vi "DataPackerDaemon.vi"(5 "Callers (Main VI name)":string, 6 "Request Debug Mode":bool, 7 "DataPacker Queue":refnum<queue>, 8 "MIDAS Sever Port":u16=12345, 9 "MIDAS Server":string="my_midas_server.domain", 10 "Override Max Event size (Data rate bytes/s). Use MIDAS Default = 0":u32) -> (0 "error out":errorcluster)   [LabVIEW 2018, in "feGEM DataPacker.lvlib"]
uses:
  feGEM DataPacker.lvlib
  DataStructures/GEM_BANK_CLUSTER_typedef.ctl
  DataStructures/GEM_DATA_cluster_typedef.ctl
  DataPacker.lvclass
  StateMachineTypeDef.ctl
  DataPacker.lvclass/DataPacker.ctl
  68ac663a-a3e9-43dc-9a45-1d254e90e99c.vi
  6484ace5-38a1-4ceb-a346-464d1fbc0e14.vi
  794d372c-62f1-4848-9cd1-c1a1182567cd.vi
  DataPacker_ConnectToMIDAS.vi/88b38ab8-c5c0-409b-a7b4-cf79df97607d.vi
  68ac663a-a3e9-43dc-9a45-1d254e90e99c.vi/471e45ec-0d50-43f9-a63f-99eed3aa29fd.vi
  6484ace5-38a1-4ceb-a346-464d1fbc0e14.vi/57d1cc16-e710-4084-af24-8dbbb67df11b.vi
  794d372c-62f1-4848-9cd1-c1a1182567cd.vi/362f5b2f-e8ea-4a71-9028-e325dbdad7c8.vi
  SendStuff/SayThisOnMIDAS.vi
  DataStructures/GEM_BANK_ARRAY_Add_Data.vi
  DataStructures/GEM_BANK_ARRAY_Flatten.vi
  ErrorTypes.ctl
  DataStructures/GEM_BANK_ARRAY.lvclass
  <vilib>/Utility/SystemLogging/NI_SystemLogging.lvlib
panel:
  out "DataPacker Queue\nUsage (%)":dbl(knob) scale=0.0..100.0
  out "CPUMEM LOAD (%)":sgl[](array[numeric])
  out "MIDAS Server IP address":string
  out "error out":errorcluster
  out "Log Client info (non fatal)":errorcluster
  out "stop":bool
  in  "stop 3":bool
  out "% Time Packing (Serializing Queued Data)":dbl(knob) scale=0.0..100.0
  out "Unsent items in queue (at shutdown)":i32
  out "MIDAS Reply":string
  out "# elements in queue":i32
  out "Connection Attempt":u32
  out "MIDAS Addresss":string
  out "MIDAS Port":u16
  out "Frontend Status":string
  out "MIDAS Buffer [for this PC] \nUsage (%)":dbl(knob) scale=0.0..100.0
  out "MIDAS Connection OK":bool
  out "Seconds since last communication with MIDAS":dbl
  out "Last Midas Handling Time (ms)":dbl
  out "Average MIDAS Processing Time (ms)":dbl(knob) scale=1.0..1000.0
  out "System Load Logging Error  (non fatal)":errorcluster
  out "Periodic Task Error (non fatal)":errorcluster
  out "This Computer Name":string
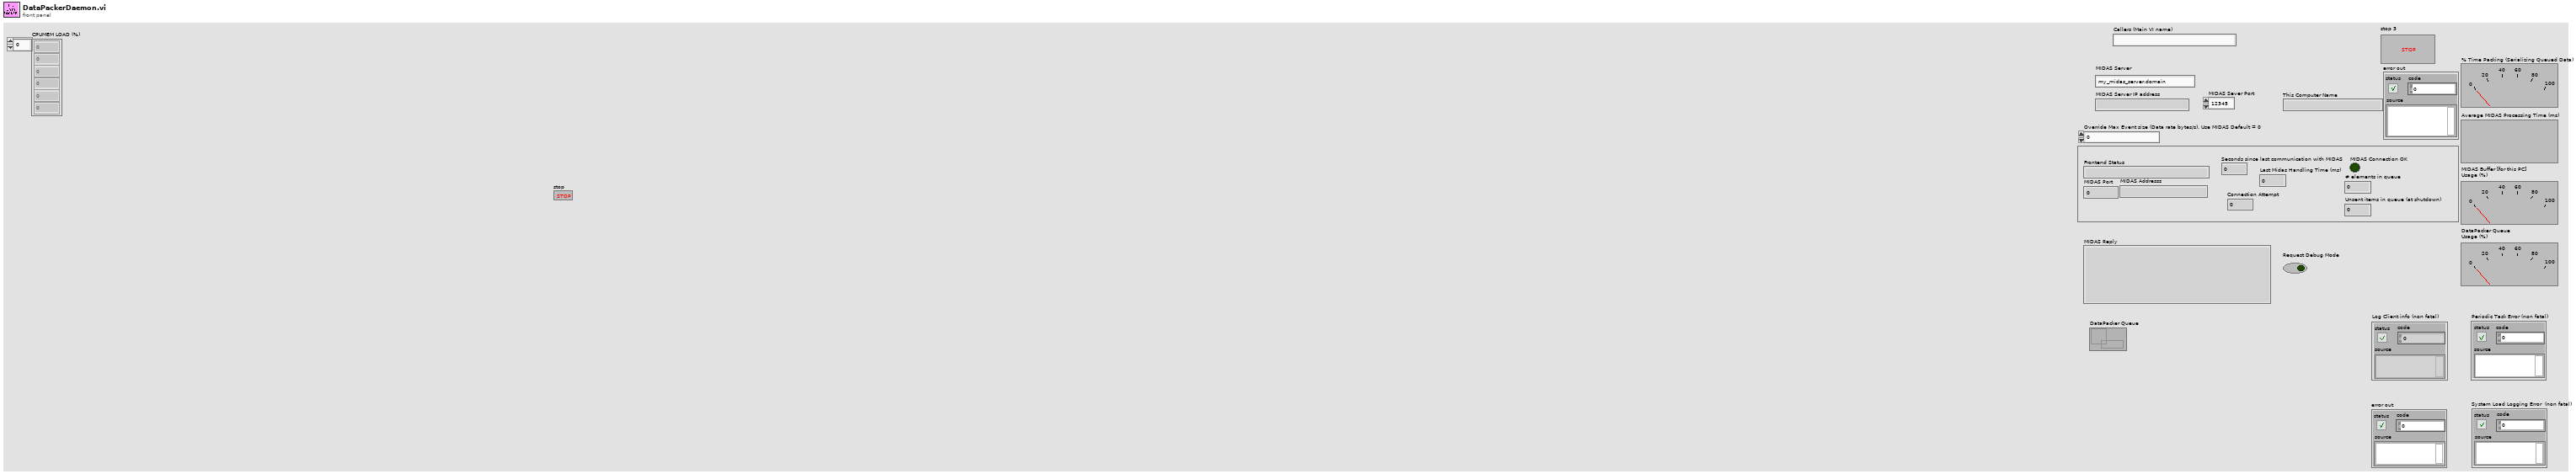
[diagram p1: front panel]
types:
  T1 = typedef "feGEM DataPacker.lvlib/StateMachineTypeDef.ctl" = enum16{"Setup", "Setup SSH", "Connect To Midas", "Get And Set Event Size", "Re-initialise", "Sleep", "BundleDataInQueue", "SerializeBundle", "SendData", "Shutdown", "HandleErrorStates"}
  T2 = typedef "feGEM DataPacker.lvlib/ErrorTypes.ctl" = i32
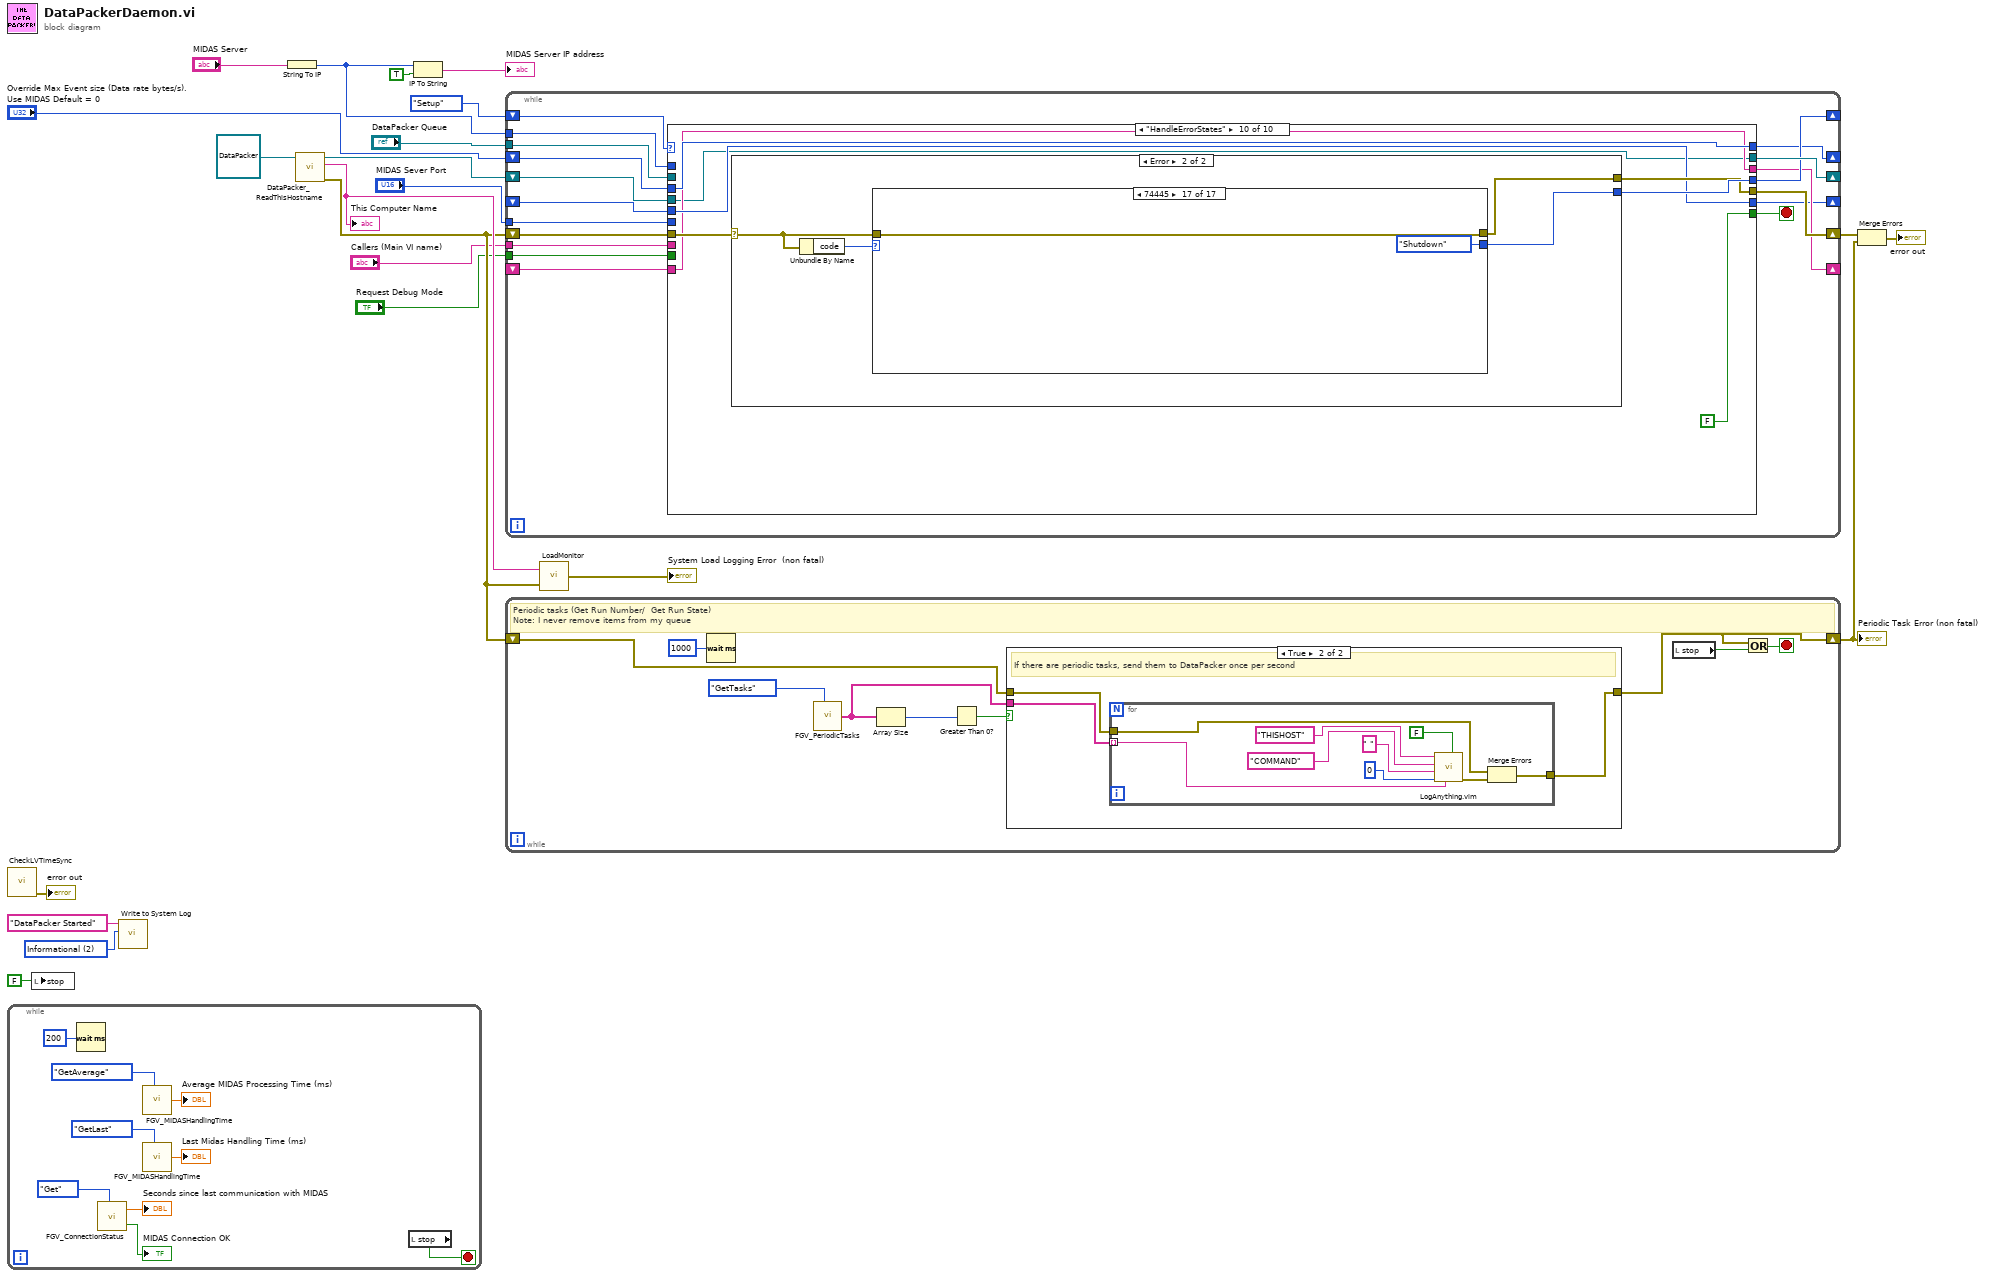
[diagram p0: block diagram]
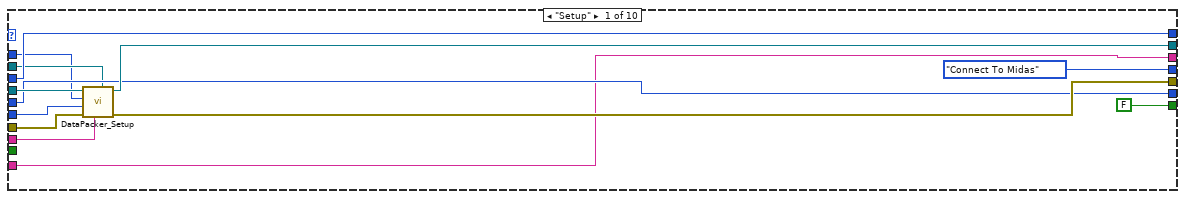
[diagram p2: hidden frame]
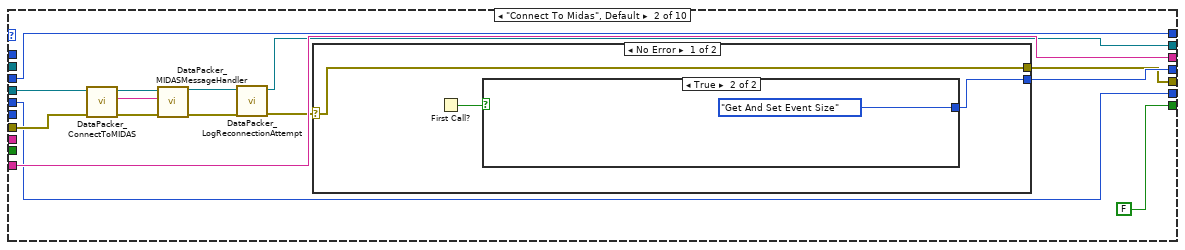
[diagram p3: hidden frame]
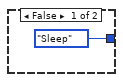
[diagram p4: hidden frame]
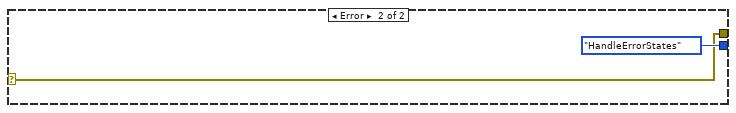
[diagram p5: hidden frame]
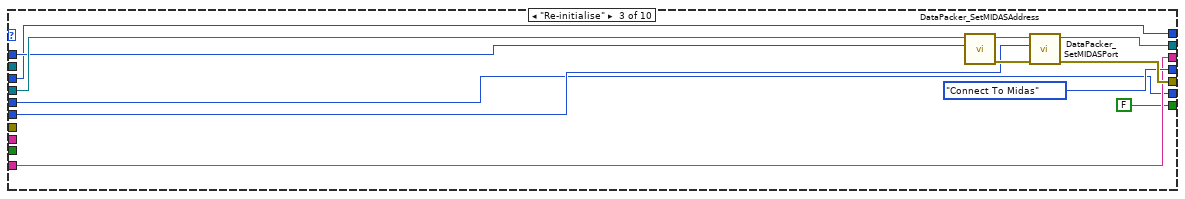
[diagram p6: hidden frame]
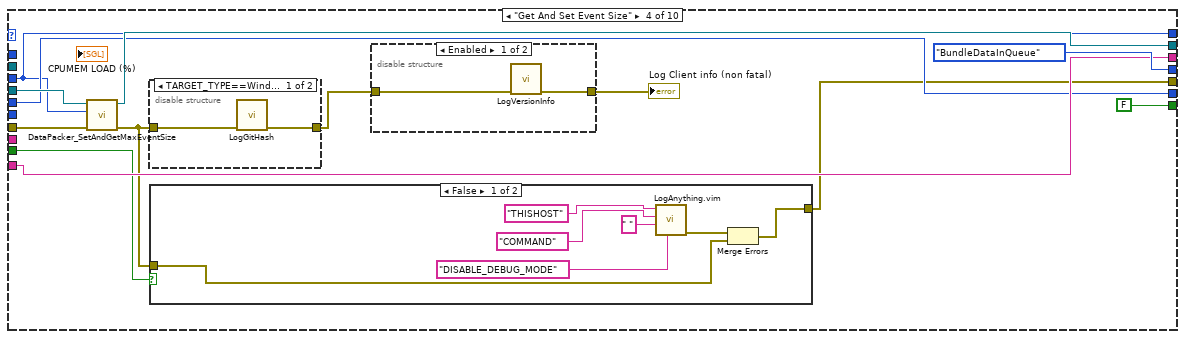
[diagram p7: hidden frame]
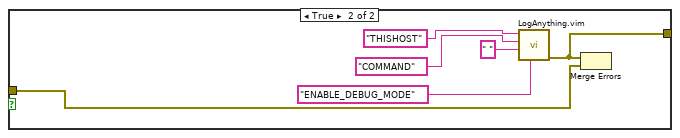
[diagram p8: hidden frame]
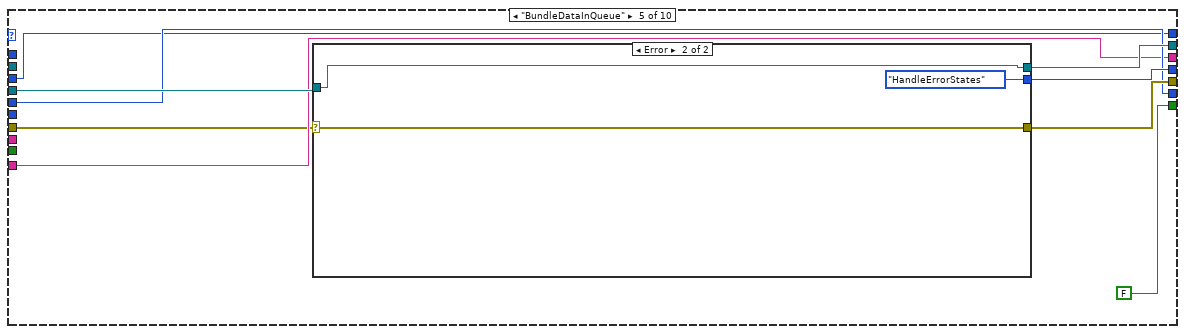
[diagram p11: hidden frame]
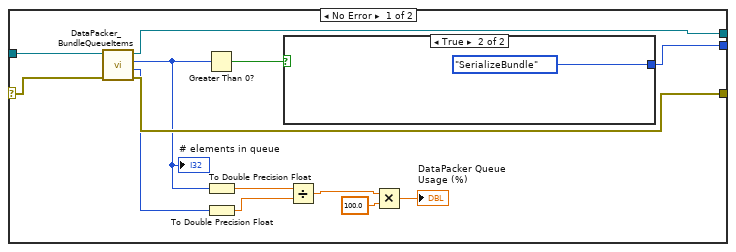
[diagram p12: hidden frame]
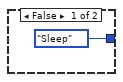
[diagram p13: hidden frame]
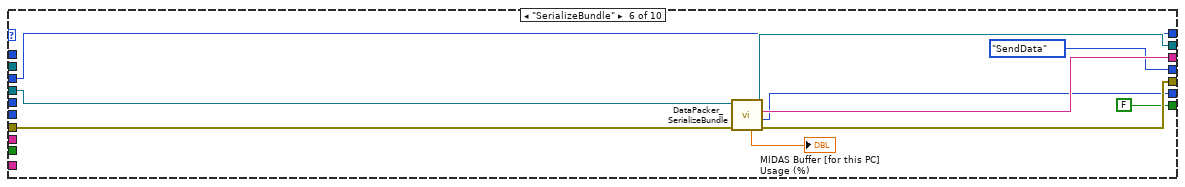
[diagram p14: hidden frame]
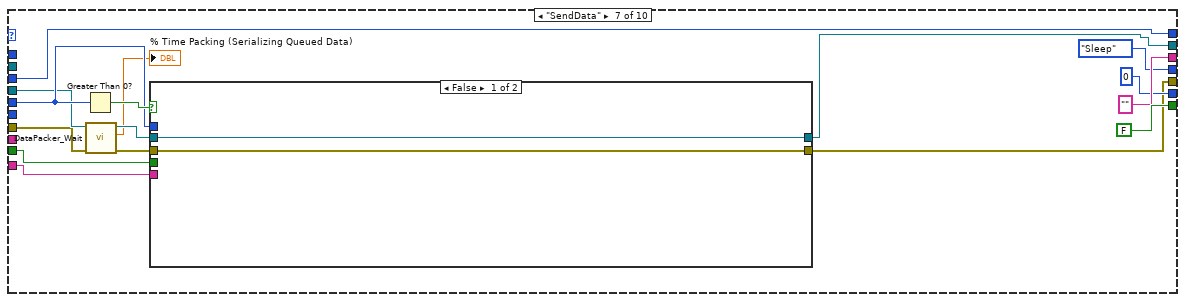
[diagram p15: hidden frame]
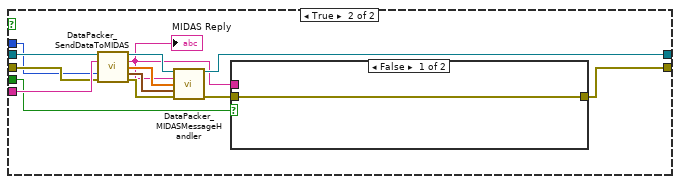
[diagram p16: hidden frame]
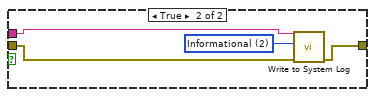
[diagram p17: hidden frame]
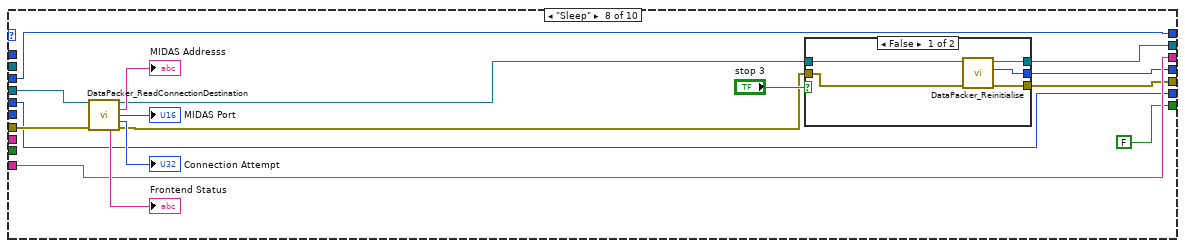
[diagram p18: hidden frame]
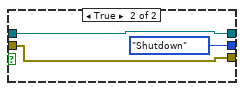
[diagram p19: hidden frame]
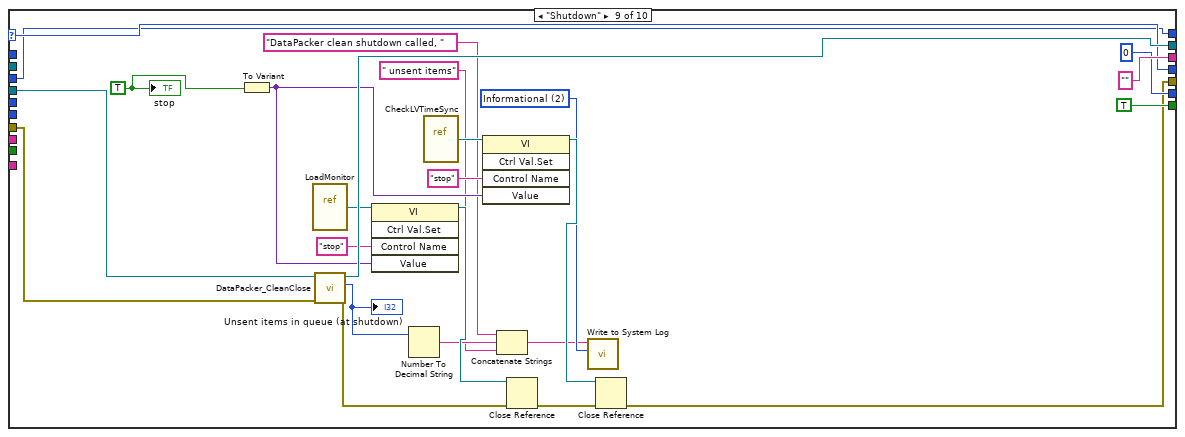
[diagram p20: hidden frame]
diagram:
  w5 = 2 items=["Error", "Warning", "Informational"] ("severity")
  n1 = call "CheckLVTimeSync.vi"() -> ("error out"=→"error out":errorcluster)  [unwired: 11 in]
  n2 = while {
    stop <- w24 stop-if-true
    n3 = Wait (ms)(milliseconds to wait=u32 200) -> ()  [unwired: 1 out]
    n4 = call "FGV_ConnectionStatus.vi"("Enum"=enum16{"Get", "Set"}."Get") -> ("Seconds since last communication with MIDAS"=→"Seconds since last communication with MIDAS":dbl, "MIDAS Connection OK"=→"MIDAS Connection OK":bool)  [unwired: 4 in]
    n5 = call "FGV_MIDASHandlingTime.vi"("Enum"=enum16{"Set", "GetLast", "GetAverage"}."GetAverage") -> ("Midas Handling Time"=→"Average MIDAS Processing Time (ms)":dbl)  [unwired: 4 in]
    n6 = call "FGV_MIDASHandlingTime.vi"("Enum"=enum16{"Set", "GetLast", "GetAverage"}."GetLast") -> ("Midas Handling Time"=→"Last Midas Handling Time (ms)":dbl)  [unwired: 4 in]
    n7 = local read "stop"() -> (w24:bool)
  }
  n8 = local write "stop"(FALSE) -> ()
  n9 = call <vilib>:"Write to System Log.vi"("severity"=w5, "message"="DataPacker Started") -> ()  [unwired: 9 in, 1 out]
  n10 = String To IP(1:"MIDAS Server") -> (0:w9:u32)
  n11 = call "DataPacker_ReadThisHostname.vi"("DataPacker in"=refnum<class "DataPacker.lvclass"> refnum ("DataPacker.lvclass")) -> ("error out"=w13:errorcluster, "This Hostname"=w21:string, "DataPacker out"=w19:refnum<class "DataPacker.lvclass">)  [unwired: 8 in]
  "This Computer Name" <- w21
  n12 = IP To String(1:TRUE ("dot notation? (F)"), 2:w9) -> (0:→"MIDAS Server IP address":string)
  n13 = while {
    shift-right: [w44] -> _
    shift-left: StateMachineTypeDef."Setup" ("Enum") -> [w47]
    shift-right: [w46] -> _
    shift-left: w19 -> [w49]
    shift-right: [w45] -> w4
    shift-left: w13 -> [w48]
    shift-right: [w42] -> _
    shift-left: _ -> [w39]
    shift-right: [w41] -> _
    shift-left: _ -> [w40]
    shift-right: [w38] -> _
    shift-left: "Override Max Event size (Data rate bytes/s). Use MIDAS Default = 0" -> [w43]
    tunnel: "MIDAS Sever Port" -> [w37]
    tunnel: "Callers (Main VI name)" -> [w36]
    tunnel: "DataPacker Queue" -> [w34]
    tunnel: w9 -> [w33]
    tunnel: "Request Debug Mode" -> [w32]
    stop <- w35 stop-if-true
    n14 = case shown="\"HandleErrorStates\"" w47 {
      selector: w47 -> [_ _ _ _ _ _ _ _ w244 _]
      tunnel: w49 -> [w60 w77 w92 w109 w137 w165 w171 w217 w250 w252]
      tunnel: w48 -> [w62 w76 _ w108 w129 w164 w170 w216 w248 w258]
      tunnel: [w58 w66 w93 w107 w135 w163 w178 w202 w249 w252] -> w46
      tunnel: [w59 w63 w94 w97 w136 w162 w173 w203 w232 w256] -> w45
      tunnel: [StateMachineTypeDef."Connect To Midas" ("Enum") w64 StateMachineTypeDef."Connect To Midas" ("Enum") StateMachineTypeDef."BundleDataInQueue" ("Enum") w134 StateMachineTypeDef."SendData" ("Enum") StateMachineTypeDef."Sleep" ("Enum") w206 w244 w257] -> w44
      tunnel: w43 -> [w56 w73 w86 w102 w130 w156 w174 w208 w243 w255]
      tunnel: [w54 w74 w88 w104 w132 w161 "" w211 "" ("SerialisedData") w253] -> w42
      tunnel: [w55 w69 w87 w103 w133 w160 0 ("Length of \nData bundle") w210 0 ("Length of \nData bundle") w254] -> w41
      tunnel: w40 -> [w55 w69 w87 w103 w133 _ w180 w210 _ w254]
      tunnel: w39 -> [w54 w74 w88 w104 w132 _ w179 w211 _ w253]
      tunnel: [FALSE FALSE FALSE FALSE FALSE FALSE FALSE FALSE TRUE FALSE] -> w35
      tunnel: [w56 w73 w86 w102 w130 w156 w174 w208 w243 w255] -> w38
      tunnel: w37 -> [w61 _ w90 _ _ _ _ _ _ _]
      tunnel: w36 -> [w57 _ _ _ _ _ _ _ _ _]
      tunnel: w34 -> [w52 _ _ _ _ _ _ _ _ _]
      tunnel: w33 -> [w50 _ w89 _ _ _ _ _ _ _]
      tunnel: w32 -> [_ _ _ w99 _ _ w166 _ _ _]
      frame "Setup" {
        n15 = call "DataPacker_Setup.vi"("DataPacker Queue"=w52, "Main VI Name"=w57, "error in (no error)"=w62, "Port To Log To"=w61, "Address to Log To"=w50, "DataPacker in"=w60) -> ("error out"=w59:errorcluster, "DataPacker out"=w58:refnum<class "DataPacker.lvclass">)  [unwired: 4 in]
      }
      frame "Connect To Midas", Default {
        n16 = call "DataPacker_ConnectToMIDAS.vi"("error in (no error)"=w76, "DataPacker in"=w77) -> ("error out"=w70:errorcluster, "MIDAS Reply"=w71:string, "DataPacker out"=w72:refnum<class "DataPacker.lvclass">)  [unwired: 7 in]
        n17 = call "DataPacker_MIDASMessageHandler.vi"("DataPacker in"=w72, "Message"=w71, "error in (no error)"=w70) -> ("DataPacker out"=w68:refnum<class "DataPacker.lvclass">, "error out"=w67:errorcluster)  [unwired: 11 in]
        n18 = call "DataPacker_LogReconnectionAttempt.vi"("error in (no error)"=w67, "DataPacker in"=w68) -> ("error out"=w65:errorcluster, "DataPacker out"=w66:refnum<class "DataPacker.lvclass">)  [unwired: 8 in]
        n19 = case shown="No Error" w65 {
          selector: w65 -> [w78 w83]
          tunnel: [w80 StateMachineTypeDef."HandleErrorStates" ("Enum")] -> w64
          tunnel: [w78 w83] -> w63
          frame No Error {
            n20 = First Call?() -> (First Call?: T/F=w79:bool)
            n21 = case shown="True" w79 {
              tunnel: [StateMachineTypeDef."Sleep" ("Enum") StateMachineTypeDef."Get And Set Event Size" ("Enum")] -> w80
              frame False {
              }
              frame True {
              }
            }
          }
          frame Error {
          }
        }
      }
      frame "Re-initialise" {
        n22 = call "DataPacker_SetMIDASAddress.vi"("Address to Log To"=w89, "DataPacker in"=w92) -> ("error out"=w95:errorcluster, "DataPacker out"=w96:refnum<class "DataPacker.lvclass">)  [unwired: 8 in]
        n23 = call "DataPacker_SetMIDASPort.vi"("error in (no error)"=w95, "Port To Log To"=w90, "DataPacker in"=w96) -> ("error out"=w94:errorcluster, "DataPacker out"=w93:refnum<class "DataPacker.lvclass">)  [unwired: 7 in]
      }
      frame "Get And Set Event Size" {
        n24 = call "DataPacker_SetAndGetMaxEventSize.vi"("error in (no error)"=w108, "Set Event Max Size"=w102, "DataPacker in"=w109) -> ("error out"=w98:errorcluster, "DataPacker out"=w107:refnum<class "DataPacker.lvclass">)  [unwired: 7 in]
        n25 = disable-structure shown="TARGET_TYPE==Windows" {
          disable-tunnel: w98 -> [w124 w125]
          disable-tunnel: [w123 w125] -> w100
          frame condition #0 (active) {
            n26 = call "LogGitHash.vi"("error in (no error)"=w124) -> ("error out"=w123:errorcluster)  [unwired: 10 in]
          }
          frame condition #1 {
          }
        }
        n27 = case shown="False" w99 {
          tunnel: w98 -> [w112 w118]
          tunnel: [w110 w117] -> w97
          frame False {
            n28 = call "LogAnything.vim"("Equipment description (32 chars)"="DISABLE_DEBUG_MODE" ("Equipment description"), "Array"=" ", "Variable Name"="COMMAND" ("Var Name"), "Category"="THISHOST") -> ("error out"=w111:errorcluster)  [unwired: 6 in, 1 out]
            n29 = Merge Errors(w111, w112) -> (w110:errorcluster)
          }
          frame True {
            n30 = call "LogAnything.vim"("Equipment description (32 chars)"="ENABLE_DEBUG_MODE" ("Equipment description"), "Array"=" ", "Variable Name"="COMMAND" ("Var Name"), "Category"="THISHOST") -> ("error out"=w117:errorcluster)  [unwired: 6 in, 1 out]
            n31 = Merge Errors(w117, w118) -> ()  [unwired: 1 out]
          }
        }
        n32 = disable-structure shown="Enabled" {
          disable-tunnel: w100 -> [w127 w128]
          disable-tunnel: [w126 w128] -> w101
          frame Enabled {
            n33 = call "LogVersionInfo.vi"("error in (no error)"=w127) -> ("error out"=w126:errorcluster)  [unwired: 10 in]
          }
          frame Disabled {
          }
        }
        "Log Client info (non fatal)" <- w101
      }
      frame "BundleDataInQueue" {
        n34 = case shown="Error" w129 {
          selector: w129 -> [w138 w154]
          tunnel: w137 -> [w150 w153]
          tunnel: [w149 w154] -> w136
          tunnel: [w148 w153] -> w135
          tunnel: [w146 StateMachineTypeDef."HandleErrorStates" ("Enum")] -> w134
          frame No Error {
            n35 = call "DataPacker_BundleQueueItems.vi"("error in (no error)"=w138, "DataPacker in"=w150) -> ("error out"=w149:errorcluster, "max queue size"=w144:i32, "# elements in queue"=w145:i32, "DataPacker out"=w148:refnum<class "DataPacker.lvclass">)  [unwired: 6 in]
            "# elements in queue" <- w145
            n36 = Greater Than 0?(x=w145) -> (x > 0?=w147:bool)
            n37 = To Double Precision Float(number=w145) -> (double precision float=w142:dbl)
            n38 = To Double Precision Float(number=w144) -> (double precision float=w143:dbl)
            n39 = case shown="True" w147 {
              tunnel: [StateMachineTypeDef."Sleep" ("Enum") StateMachineTypeDef."SerializeBundle" ("Enum")] -> w146
              frame False {
              }
              frame True {
              }
            }
            n40 = Divide(x=w142, y=w143) -> (x/y=w141:dbl)
            n41 = Multiply(x=w141, y=100.0) -> (x*y=→"DataPacker Queue\nUsage (%)":dbl)
          }
          frame Error {
          }
        }
      }
      frame "SerializeBundle" {
        n42 = call "DataPacker_SerializeBundle.vi"("error in (no error)"=w164, "DataPacker in"=w165) -> ("error out"=w162:errorcluster, "Length of \nData bundle"=w160:i32, "SerialisedData"=w161:string, "DataPacker out"=w163:refnum<class "DataPacker.lvclass">, "MIDAS Buffer \n[for this PC] \nUsage (%)"=→"MIDAS Buffer [for this PC] \nUsage (%)":dbl)  [unwired: 5 in]
      }
      frame "SendData" {
        n43 = Greater Than 0?(x=w180) -> (x > 0?=w181:bool)
        n44 = call "DataPacker_Wait.vi"("error in (no error)"=w170, "DataPacker in"=w171) -> ("error out"=w169:errorcluster, "% Time Packing (Serializing Queued Data)"=→"% Time Packing (Serializing Queued Data)":dbl, "DataPacker out"=w168:refnum<class "DataPacker.lvclass">)  [unwired: 7 in]
        n45 = case shown="False" w181 {
          tunnel: w180 -> [_ w190]
          tunnel: w179 -> [_ w194]
          tunnel: w168 -> [w183 w192]
          tunnel: w169 -> [w182 w191]
          tunnel: [w182 w185] -> w173
          tunnel: [w183 w193] -> w178
          tunnel: w166 -> [_ w184]
          frame False {
          }
          frame True {
            n46 = call "DataPacker_SendDataToMIDAS.vi"("DataPacker in"=w192, "data in"=w194, "data in length"=w190, "error in (no error)"=w191) -> ("DataPacker out"=w195:refnum<class "DataPacker.lvclass">, "MIDAS Reply"=w187:string, "Send Time, Recieve Time"=w188:dbl[], "MIDAS Comm finished"=w189:timestamp, "error out"=w196:errorcluster)  [unwired: 7 in]
            "MIDAS Reply" <- w187
            n47 = call "DataPacker_MIDASMessageHandler.vi"("DataPacker in"=w195, "Message"=w187, "Array"=w188, "MIDAS Comm finish time"=w189, "error in (no error)"=w196) -> ("DataPacker out"=w193:refnum<class "DataPacker.lvclass">, "error out"=w186:errorcluster)  [unwired: 9 in]
            n48 = case shown="False" w184 {
              tunnel: w187 -> [_ w201]
              tunnel: w186 -> [w197 w199]
              tunnel: [w197 w198] -> w185
              frame False {
              }
              frame True {
                w200 = 2 items=["Error", "Warning", "Informational"] ("severity")
                n49 = call <vilib>:"Write to System Log.vi"("error in (no error)"=w199, "severity"=w200, "message"=w201) -> ("error out"=w198:errorcluster)  [unwired: 8 in]
              }
            }
          }
        }
      }
      frame "Sleep" {
        n50 = call "DataPacker_ReadConnectionDestination.vi"("DataPacker in"=w217, "error in (no error)"=w216) -> ("DataPacker out"=w204:refnum<class "DataPacker.lvclass">, "MIDAS Addresss"=→"MIDAS Addresss":string, "MIDAS Port"=→"MIDAS Port":u16, "Connection Attempt"=→"Connection Attempt":u32, "Frontend Status"=→"Frontend Status":string, "error out"=w205:errorcluster)  [unwired: 8 in]
        n51 = case shown="False" "stop 3" {
          tunnel: [w218 StateMachineTypeDef."Shutdown" ("Enum")] -> w206
          tunnel: w205 -> [w222 w223]
          tunnel: w204 -> [w221 w224]
          tunnel: [w220 w223] -> w203
          tunnel: [w219 w224] -> w202
          frame False {
            n52 = call "DataPacker_Reinitialise.vi"("error in (no error)"=w222, "DataPacker in"=w221) -> ("error out"=w220:errorcluster, "Next State"=w218:T1, "DataPacker out"=w219:refnum<class "DataPacker.lvclass">)  [unwired: 7 in]
          }
          frame True {
          }
        }
      }
      frame "Shutdown" {
        w231 = 2 items=["Error", "Warning", "Informational"] ("severity")
        w239 = TRUE
        n53 = To Variant(anything=w239) -> (Variant=w236:variant)
        n54 = vi-ref "LoadMonitor.vi"() -> (w241:refnum<vi>)
        n55 = call "DataPacker_CleanClose.vi"("error in (no error)"=w248, "DataPacker in"=w250) -> ("error out"=w234:errorcluster, "Unsent items in queue"=w230:i32, "DataPacker out"=w249:refnum<class "DataPacker.lvclass">)  [unwired: 7 in]
        "Unsent items in queue (at shutdown)" <- w230
        n56 = invoke class="VI" method="Ctrl Val.Set"(reference=w241, "Control Name"="stop", "Value"=w236) -> (reference out=w242:refnum<vi>)  [unwired: 2 in, 4 out]
        n57 = Number To Decimal String(number=w230) -> (decimal integer string=w228:string)  [unwired: 1 in]
        n58 = vi-ref "CheckLVTimeSync.vi"() -> (w238:refnum<vi>)
        n59 = invoke class="VI" method="Ctrl Val.Set"(reference=w238, "Control Name"="stop", "Value"=w236) -> (reference out=w235:refnum<vi>)  [unwired: 2 in, 4 out]
        n60 = Concatenate Strings("DataPacker clean shutdown called, " ("message"), w228, " unsent items" ("string")) -> (w226:string)
        n61 = Close Reference(reference=w242, error in (no error)=w234) -> (error out=w233:errorcluster)
        n62 = call <vilib>:"Write to System Log.vi"("severity"=w231, "message"=w226) -> ()  [unwired: 9 in, 1 out]
        n63 = Close Reference(reference=w235, error in (no error)=w233) -> (error out=w232:errorcluster)
        "stop" <- w239
      }
      frame "HandleErrorStates" {
        n64 = case shown="Error" w258 {
          selector: w258 -> [w259 w261]
          tunnel: [StateMachineTypeDef."Sleep" ("Enum") w263] -> w257
          tunnel: [w259 w262] -> w256
          frame No Error {
          }
          frame Error {
            n65 = Unbundle By Name(w261) -> ("code"=w264:i32)
            n66 = case shown="74445" w264 {
              tunnel: [StateMachineTypeDef."Sleep" ("Enum") StateMachineTypeDef."Re-initialise" ("Enum") StateMachineTypeDef."Re-initialise" ("Enum") StateMachineTypeDef."Re-initialise" ("Enum") StateMachineTypeDef."Re-initialise" ("Enum") StateMachineTypeDef."Re-initialise" ("Enum") StateMachineTypeDef."Re-initialise" ("Enum") StateMachineTypeDef."Re-initialise" ("Enum") StateMachineTypeDef."Re-initialise" ("Enum") StateMachineTypeDef."Re-initialise" ("Enum") StateMachineTypeDef."Re-initialise" ("Enum") StateMachineTypeDef."Re-initialise" ("Enum") StateMachineTypeDef."Re-initialise" ("Enum") StateMachineTypeDef."Re-initialise" ("Enum") StateMachineTypeDef."Shutdown" ("Enum") StateMachineTypeDef."Shutdown" ("Enum") StateMachineTypeDef."Shutdown" ("Enum")] -> w263
              tunnel: [w265 _ _ _ _ _ _ _ _ _ _ _ _ _ w280 w282 w285] -> w262
              tunnel: w261 -> [w265 _ _ _ _ _ _ _ _ _ _ _ _ _ w280 w282 w285]
              frame 0, Default {
              }
              frame 1 {
                # "Unknown error type... but its bad?"
              }
              frame 55 {
                # "UDP / TCP Errors"
              }
              frame 56 {
                # "UDP / TCP Errors"
              }
              frame 57 {
                # "UDP / TCP Errors"
              }
              frame 58 {
                # "UDP / TCP Errors"
              }
              frame 59 {
                # "UDP / TCP Errors"
              }
              frame 60 {
                # "UDP / TCP Errors"
              }
              frame 61 {
                # "UDP / TCP Errors"
              }
              frame 62 {
                # "UDP / TCP Errors"
              }
              frame 63 {
                # "UDP / TCP Errors"
              }
              frame 64 {
                # "UDP / TCP Errors"
              }
              frame 65 {
                # "UDP / TCP Errors"
              }
              frame 66 {
                # "UDP / TCP Errors"
              }
              frame 74443 {
                n67 = disable-structure shown="Disabled" {
                  frame Disabled {
                    (unwired) T2 74443 items=["No Error"=0, "Network: mgNotSupported"=53, "Network: ncBadAddressErr"=54, "Network: ncInProgressErr"=55, "Network: ncTimeOutErr"=56, "Network: ncBusyErr"=57, "Network: ncNotSupportedErr"=58, "Network: ncNetErr"=59, "Network: ncAddrInUseErr"=60, "Network: ncSysOutOfMemErr"=61, "Network: ncSysOutOfMemErr"=62, "Network: ncConnRefusedErr"=63, "Network: ncAlreadyConnectedErr"=65, "Network: ncConnClosedErr"=66, "MIDAS buffer overflow!"=74443, "LVBANK CORRUPTION"=74444] ("Ring")
                  }
                  frame Enabled {
                  }
                }
              }
              frame 74444 {
                n68 = disable-structure shown="Disabled" {
                  frame Disabled {
                    (unwired) T2 74444 items=["No Error"=0, "Network: mgNotSupported"=53, "Network: ncBadAddressErr"=54, "Network: ncInProgressErr"=55, "Network: ncTimeOutErr"=56, "Network: ncBusyErr"=57, "Network: ncNotSupportedErr"=58, "Network: ncNetErr"=59, "Network: ncAddrInUseErr"=60, "Network: ncSysOutOfMemErr"=61, "Network: ncSysOutOfMemErr"=62, "Network: ncConnRefusedErr"=63, "Network: ncAlreadyConnectedErr"=65, "Network: ncConnClosedErr"=66, "LVBANK CORRUPTION"=74444] ("Ring")
                  }
                  frame Enabled {
                  }
                }
              }
              frame 74445 {
              }
            }
          }
        }
      }
    }
  }
  n69 = while {
    shift-right: [w289] -> w3
    shift-left: w13 -> [w290]
    stop <- w288 stop-if-true
    # "Periodic tasks (Get Run Number/  Get Run State)\nNote: I never remove items from my queue"
    n70 = Wait (ms)(milliseconds to wait=u32 1000) -> ()  [unwired: 1 out]
    n71 = call "FGV_PeriodicTasks.vi"("Task"=enum16{"AddTask", "GetTasks", "ClearTasks"}."GetTasks" ("Enum")) -> ("Tasks"=w291:string[])  [unwired: 4 in]
    n72 = Array Size(array=w291) -> (size(s)=w292:i32)
    n73 = Greater Than 0?(x=w292) -> (x > 0?=w293:bool)
    n74 = case shown="True" w293 {
      tunnel: w291 -> [_ w298]
      tunnel: w290 -> [w295 w297]
      tunnel: [w295 w296] -> w289
      frame False {
      }
      frame True {
        # "If there are periodic tasks, send them to DataPacker once per second"
        n75 = for {
          tunnel: w298 -> [w299] mode=indexing
          tunnel: w297 -> [w307]
          tunnel: [w306] -> w296
          n76 = call "LogAnything.vim"("Skip ODB on the way to \nhistories (fast, but no ALARMS possible)"=FALSE ("Get Default History Period from MIDAS\n(optional)"), "Equipment description (32 chars)"=w299, "Period to update history plots (seconds)\nUnset (65535) = Use MIDAS default in ODB\n0 = Record but do not put in histories"=0 ("Rate to update history plots"), "Array"=" ", "Variable Name"="COMMAND" ("Var Name"), "Category"="THISHOST") -> ("error out"=w302:errorcluster)  [unwired: 4 in, 1 out]
          n77 = Merge Errors(w307, w302) -> (w306:errorcluster)
        }
      }
    }
    n78 = local read "stop"() -> (w287:bool)
    n79 = Or(x=w289, y=w287) -> (x .or. y?=w288:bool)
  }
  "Periodic Task Error (non fatal)" <- w3
  n80 = call "LoadMonitor.vi"("error out"=w13, "hostname"=w21) -> ("error IO"=→"System Load Logging Error  (non fatal)":errorcluster)
  n81 = Merge Errors(w4, w3) -> (→"error out":errorcluster)
